vi "Tx Write Single Point.vi"(8 "error in (no error)":errorcluster, 10 "Outgoing data":dbl[](array[numeric]), 11 "Tx Event In":T1) -> (0 "error out":errorcluster, 3 "Tx Event Out":T1)   [LabVIEW 2020, in "985x Support Addon Engine.lvlib"]
uses:
  985x Support Addon Engine.lvlib
  Types/Tx Event Session.ctl
  Types/FPGA Refnum.ctl
  <vilib>/xnet/xnet.llb/XNET Convert (Signal to Frame CAN).vi
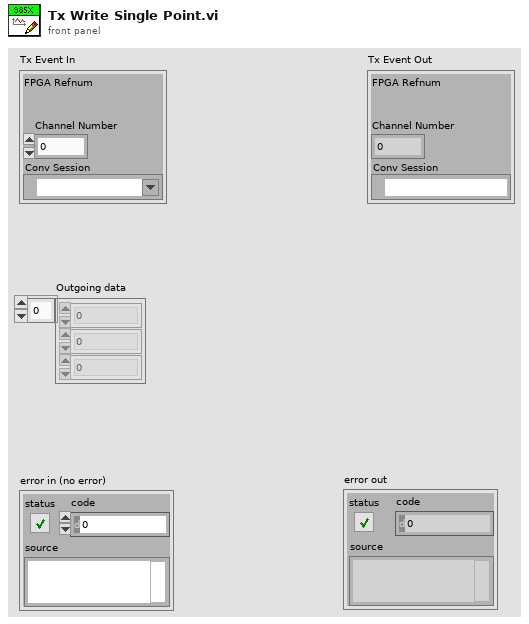
[diagram p1: front panel]
types:
  T1 = typedef "985x Support Addon Engine.lvlib/Tx Event Session.ctl" = cluster{"FPGA Refnum":T2, "Channel Number":u32, "Conv Session":refnum<k21>}
  T2 = typedef "985x Support Addon Engine.lvlib/FPGA Refnum.ctl" = refnum<k20>
  T3 = typedef "XNET Frame CAN.ctl" = cluster{"timestamp":timestamp, "payload":u8[], "identifier":u32, "type":T4, "extended?":bool, "echo?":bool}
  T4 = typedef "XNET Frame Type CAN.ctl" = u8
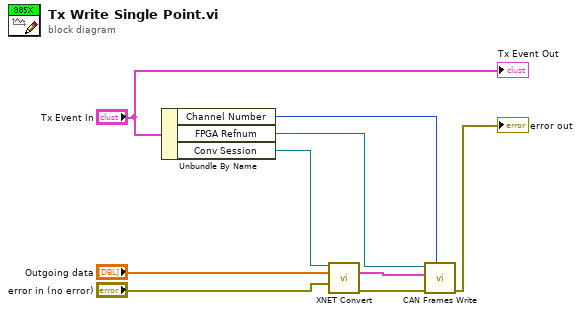
[diagram p0: block diagram]
diagram:
  n1 = Unbundle By Name("Tx Event In") -> ("Channel Number"=w1:u32, "FPGA Refnum"=w2:T2, "Conv Session"=w3:refnum<k21>)
  n2 = call-poly <vilib>:"XNET Convert.vi"("session in"=w3, "signal data"="Outgoing data", "error in (no error)"="error in (no error)") -> ("frame data"=w5:T3[], "error out"=w4:errorcluster)  [unwired: 11 out]
  n3 = call "CAN Frames Write.vi"("Channel Number"=w1, "error in (no error)"=w4, "Frames"=w5, "FPGA Refnum"=w2) -> ("error out"=→"error out":errorcluster)  [unwired: 7 in]
  "Tx Event Out" <- "Tx Event In"
